vi "error 5101.vi"() -> (0 "error out":errorcluster)   [LabVIEW 2024]
uses:
  <vilib>/Utility/error.llb/Error Cluster From Error Code.vi
  <vilib>/ErrorRing/Error Ring.xnode
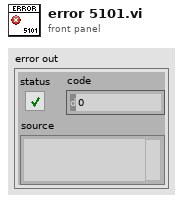
[diagram p1: front panel]
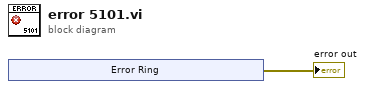
[diagram p0: block diagram]
diagram:
  n1 = xnode "Error Ring"() -> ("error out"=→"error out":errorcluster)
